vi "Error_2layerOutX_1layerOutX.vi"(1 "Array_target_ox":fxp<+/-,32,8>[](array[numeric]), 2 "Array_Out_ox":fxp<+/-,32,8>[](array[numeric]), 3 "Array_2layer_Weights_at_Index_hx":fxp<+/-,32,8>[](array[numeric])) -> (0 "Err_outX":fxp<+/-,32,8>)   [LabVIEW 2016]
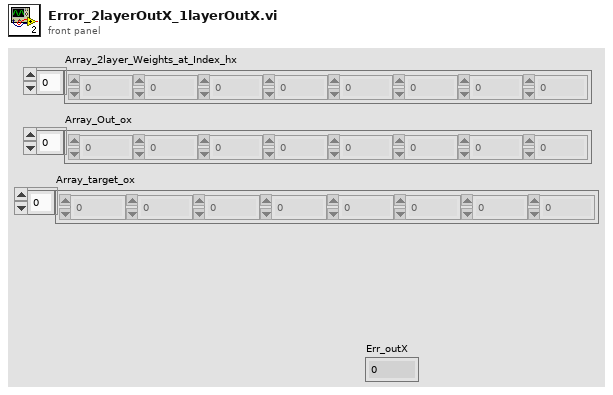
[diagram p1: front panel]
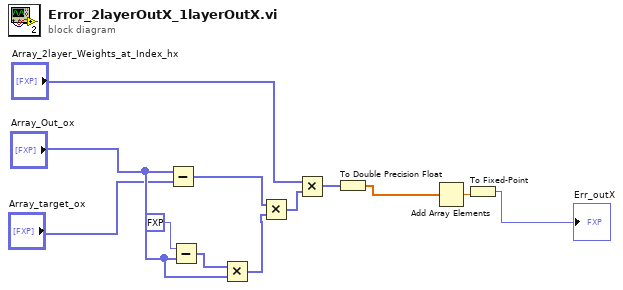
[diagram p0: block diagram]
diagram:
  n1 = Subtract(x="Array_Out_ox", y="Array_target_ox") -> (x-y=w7:fxp<+/-,33,9>[])
  n2 = Subtract(x=fxp<+,32,8> 1.0, y="Array_Out_ox") -> (x-y=w11:fxp<+/-,34,10>[])
  n3 = Multiply(x=w11, y="Array_Out_ox") -> (x*y=w6:fxp<+/-,32,8>[])
  n4 = Multiply(x=w7, y=w6) -> (x*y=w5:fxp<+/-,64,16>[])
  n5 = Multiply(x="Array_2layer_Weights_at_Index_hx", y=w5) -> (x*y=w4:fxp<+/-,32,8>[])
  n6 = To Double Precision Float(number=w4) -> (double precision float=w3:dbl[])
  n7 = Add Array Elements(numeric array=w3) -> (sum=w2:dbl)
  n8 = To Fixed-Point(number=w2) -> (fixed-point=→"Err_outX":fxp<+/-,32,8>)  [unwired: 1 in]
